vi "MicroPVHTML100_3.vi"(7 "Chaîne en entrée":string, 8 "errin":errorcluster caption="entrée d'erreur (pas d'erreur)", 10 "Chemin du fichier":path, 11 "Chemin du fichier 2":path) -> (0 "sortie d'erreur":errorcluster, 1 "Booléen":bool, 2 "Chaîne en sortie":string, 3 "nombre de PASS":i32)   [LabVIEW 2020]
uses:
  SubVi/Param_Stack.vi
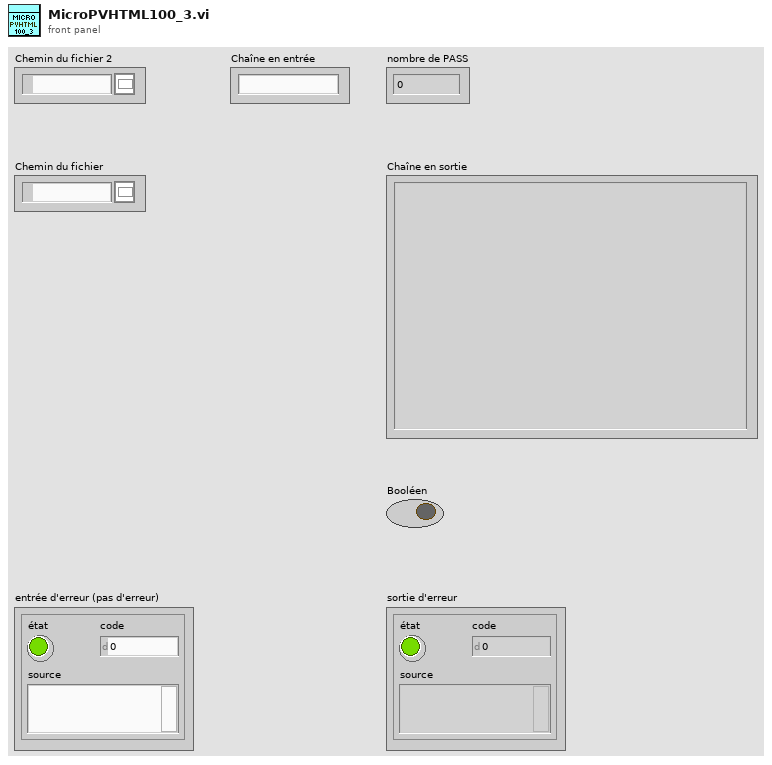
[diagram p1: front panel]
types:
  T1 = enum16{"open", "replace", "create", "open or create", "replace or create", "replace or create with confirmation"}
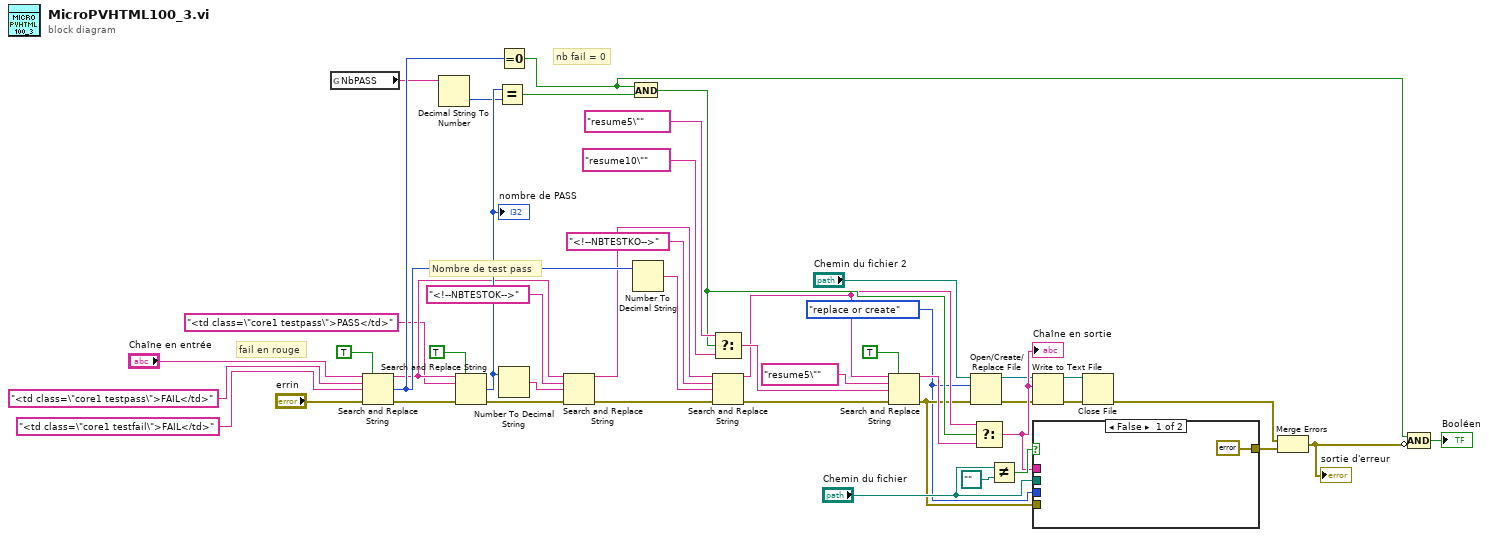
[diagram p0: block diagram]
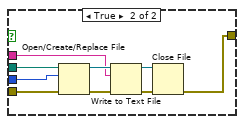
[diagram p2: hidden frame]
diagram:
  w24 = T1."replace or create" ("opération (0 : open)")
  # "nb fail = 0"
  # "Nombre de test pass"
  # "fail en rouge"
  n1 = global read "Param_Stack.vi" "NbPASS"() -> (w2:string)
  n2 = Search and Replace String(replace all?=TRUE ("tout remplacer ? (F)"), input string="Chaîne en entrée", search string="<td class=\"core1 testpass\">FAIL</td>" ("chaîne recherchée"), replace string="<td class=\"core1 testfail\">FAIL</td>" ("chaîne de remplacement (\"\")"), error in="errin") -> (result string=w23:string, number of replacements=w25:i32, error out=w13:errorcluster)  [unwired: 3 in, 1 out]
  n3 = Decimal String To Number(string=w2) -> (number=w1:i32)  [unwired: 2 in, 1 out]
  n4 = Search and Replace String(replace all?=TRUE ("tout remplacer ? (F)"), input string=w23, search string="<td class=\"core1 testpass\">PASS</td>" ("chaîne recherchée"), error in=w13) -> (number of replacements=w39:i32, error out=w17:errorcluster)  [unwired: 4 in, 2 out]
  "nombre de PASS" <- w39
  n5 = Equal?(x=w39, y=w1) -> (x = y?=w41:bool)
  n6 = Equal To 0?(x=w25) -> (x = 0?=w40:bool)
  n7 = Number To Decimal String(number=w39) -> (decimal integer string=w21:string)  [unwired: 1 in]
  n8 = Search and Replace String(input string=w23, search string="<!--NBTESTOK-->" ("chaîne recherchée"), replace string=w21, error in=w17) -> (result string=w16:string, error out=w18:errorcluster)  [unwired: 4 in, 2 out]
  n9 = And(x=w40, y=w41) -> (x .and. y?=w42:bool)
  n10 = Number To Decimal String(number=w25) -> (decimal integer string=w22:string)  [unwired: 1 in]
  n11 = Select(t="resume5\"", s=w42, f="resume10\"") -> (s? t:f=w45:string)
  n12 = Search and Replace String(input string=w16, search string="<!--NBTESTKO-->" ("chaîne recherchée"), replace string=w22, error in=w18) -> (result string=w31:string, error out=w26:errorcluster)  [unwired: 4 in, 2 out]
  n13 = Search and Replace String ("Rechercher et remplacer une chaîne")(replace all?=TRUE ("tout remplacer ? (F)"), input string=w31, search string="resume5\"", replace string=w45, error in=w26) -> (result string=w30:string, error out=w27:errorcluster)  [unwired: 3 in, 2 out]
  n14 = Open/Create/Replace File(file path (use dialog)="Chemin du fichier 2", error in=w27, operation (0:open)=w24) -> (refnum out=w6:refnum<file>, error out=w4:errorcluster)  [unwired: 3 in, 1 out]
  n15 = Select(t=w31, s=w42, f=w30) -> (s? t:f=w29:string)
  "Chaîne en sortie" <- w29
  n16 = Not Equal?(x="Chemin du fichier", y=path "") -> (x != y?=w36:bool)
  n17 = Write to Text File(file (use dialog)=w6, text=w29, error in=w4) -> (refnum out=w5:refnum<file>, error out=w3:errorcluster)  [unwired: 1 in, 1 out]
  n18 = case shown="False" w36 {
    tunnel: w24 -> [_ w52]
    tunnel: "Chemin du fichier" -> [_ w51]
    tunnel: w27 -> [_ w50]
    tunnel: w29 -> [_ w49]
    tunnel: [errorcluster {"status"=FALSE, "code"=0, "source"=""} ("error out") w48] -> w32
    frame False {
    }
    frame True {
      n19 = Open/Create/Replace File(file path (use dialog)=w51, error in=w50, operation (0:open)=w52) -> (refnum out=w53:refnum<file>, error out=w55:errorcluster)  [unwired: 3 in, 1 out]
      n20 = Write to Text File(file (use dialog)=w53, text=w49, error in=w55) -> (refnum out=w54:refnum<file>, error out=w56:errorcluster)  [unwired: 1 in, 1 out]
      n21 = Close File(refnum=w54, error in=w56) -> (error out=w48:errorcluster)  [unwired: 1 out]
    }
  }
  n22 = Close File(refnum=w5, error in=w3) -> (error out=w33:errorcluster)  [unwired: 1 out]
  n23 = Merge Errors(w33, w32) -> (w34:errorcluster)
  "sortie d'erreur" <- w34
  n24 = Compound Arithmetic op=AND ("Opérateur arithmétique")(w40, invert w34) -> (→"Booléen":bool)
